vi "GetState.vi"(6 "error in (no error)":errorcluster, 7 "Calibrate?":bool, 8 "IMU Channel":tag="A/I2C", 9 "LIDAR Channel":tag="B/I2C") -> (0 "error out":errorcluster, 1 "Height":dbl, 2 "Angular Velocity":dbl[](array[numeric]), 3 "imu accel":i16[](array[numeric]))   [LabVIEW 2017]
uses:
  <vilib>/Analysis/baseanly.llb/Mean (DBL).vi
  <vilib>/Analysis/NI_AALBase.lvlib
panel:
  out "error out 2":errorcluster
  out "Acceleration":dbl[](array[numeric])
  in  "Acceleration Factor (experimentally determined)":dbl format="%#_13g"
  out "MyRIO Acceleration":dbl[](array[numeric])
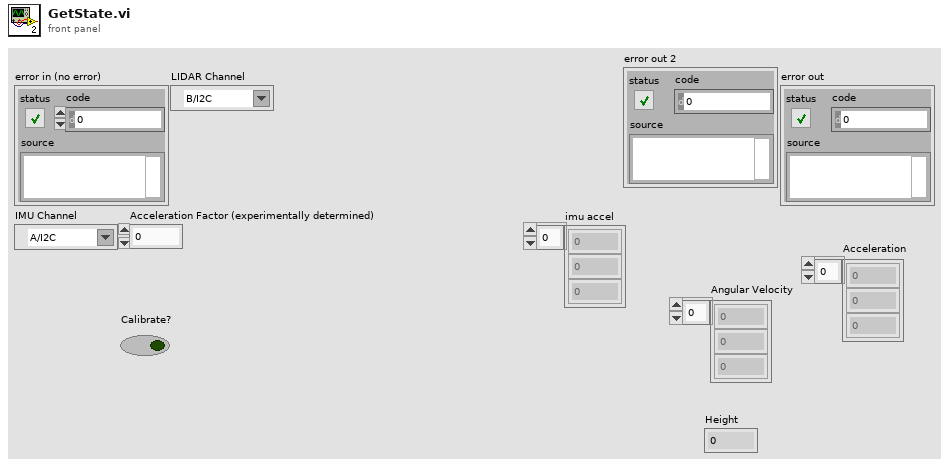
[diagram p1: front panel]
types:
  T1 = cluster{"X-axis":i16, "Y-axis":i16, "Z-axis":i16}
  T2 = cluster{"X-Axis":dbl, "Y-Axis":dbl, "Z-Axis":dbl}
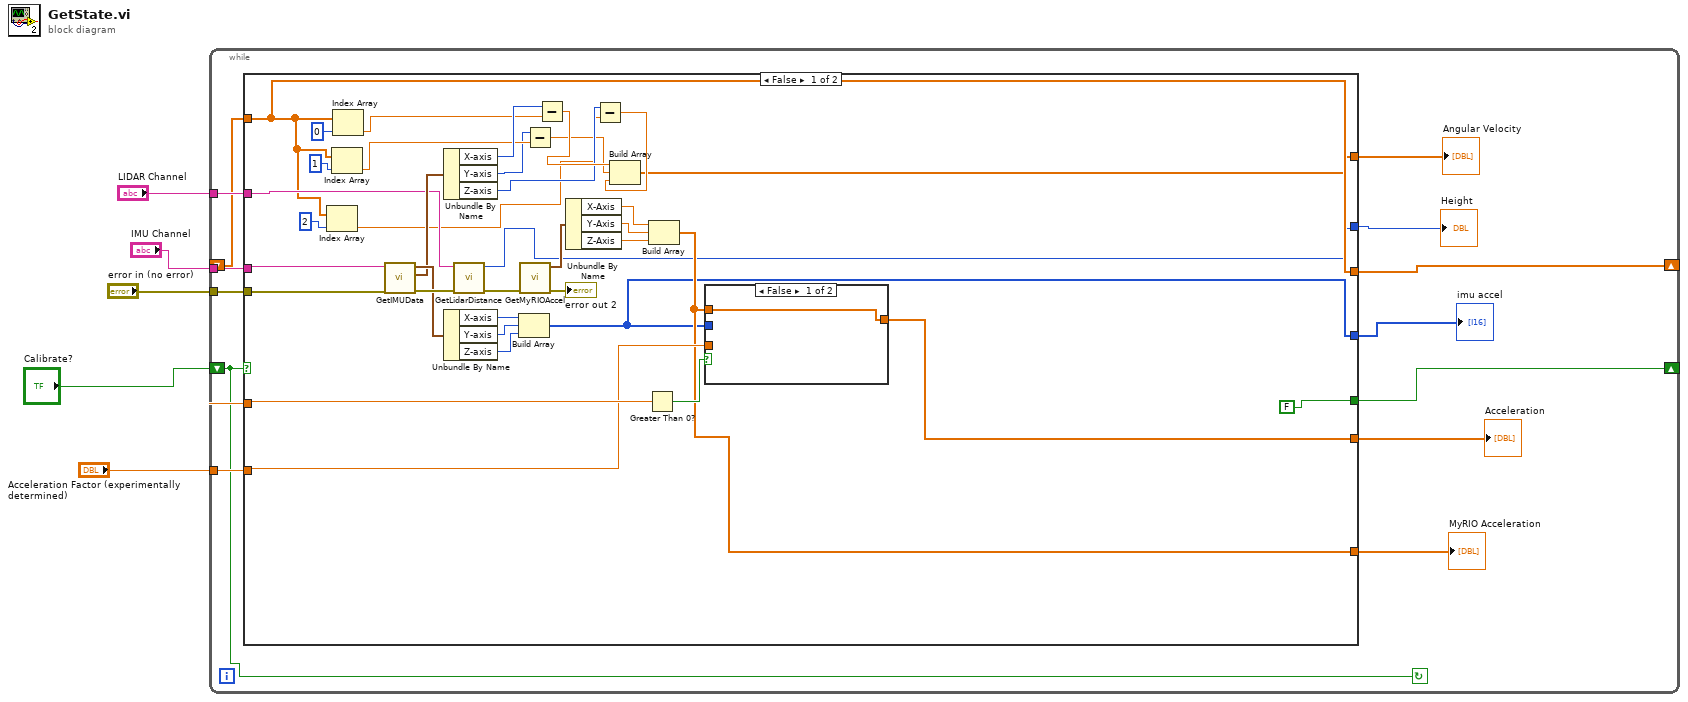
[diagram p0: block diagram]
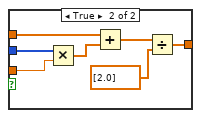
[diagram p2: hidden frame]
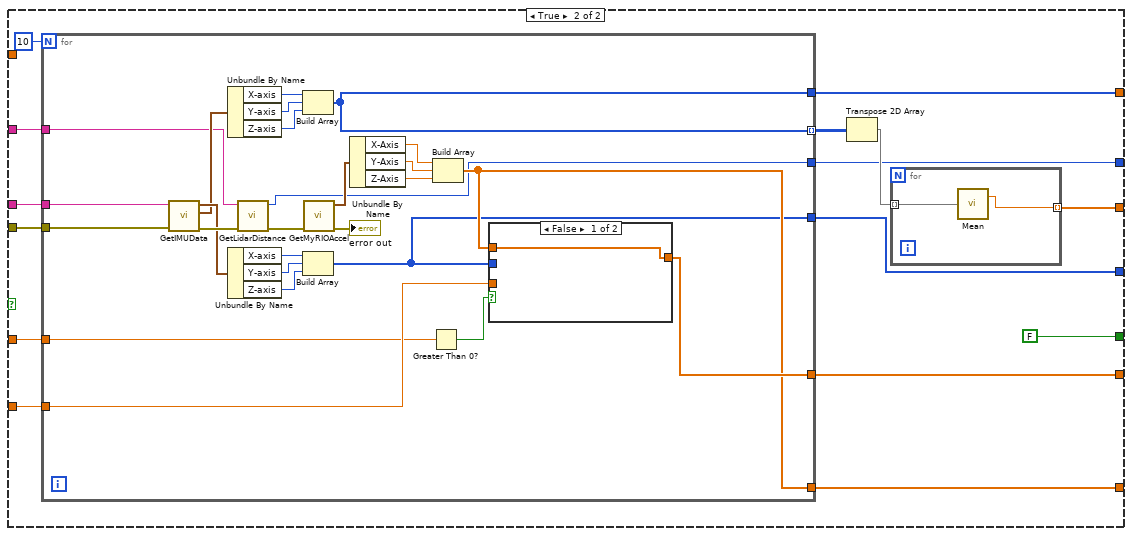
[diagram p3: hidden frame]
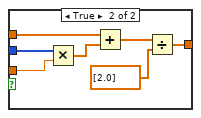
[diagram p4: hidden frame]
diagram:
  n1 = while {
    tunnel: "error in (no error)" -> [w18]
    tunnel: "IMU Channel" -> [w17]
    tunnel: "LIDAR Channel" -> [w16]
    tunnel: "Acceleration Factor (experimentally determined)" -> [w15]
    shift-right: [w14] -> _
    shift-left: "Calibrate?" -> [w13]
    shift-right: [w12] -> _
    shift-left: _ -> [w11]
    stop <- w13 continue-if-true
    n2 = case shown="False" w13 {
      tunnel: w18 -> [w40 w78]
      tunnel: w17 -> [w41 w77]
      tunnel: w16 -> [w42 w76]
      tunnel: w15 -> [w38 w75]
      tunnel: w15 -> [w39 w74]
      tunnel: [FALSE FALSE] -> w14
      tunnel: [w25 w69] -> w12
      tunnel: w11 -> [w25 _]
      tunnel: [w20 w68] -> w10
      tunnel: [w23 w67] -> w9
      tunnel: [w22 w66] -> w8
      tunnel: [w21 w65] -> w7
      tunnel: [w19 w64] -> w6
      frame False {
        n3 = Index Array(array=w25, index=2) -> (element=w28:dbl)
        n4 = Index Array(array=w25, index=1) -> (element=w31:dbl)
        n5 = Index Array(array=w25, index=0) -> (element=w35:dbl)
        n6 = call "GetIMUData.vi"("error in (no error)"=w40, "Channel Name"=w41) -> ("error out"=w55:errorcluster, "GyroData"=w50:T1, "AccelData"=w51:T1)  [unwired: 7 in]
        n7 = Unbundle By Name(w50) -> ("X-axis"=w36:i16, "Y-axis"=w30:i16, "Z-axis"=w29:i16)
        n8 = Unbundle By Name(w51) -> ("X-axis"=w46:i16, "Y-axis"=w45:i16, "Z-axis"=w44:i16)
        n9 = call "GetLidarDistance.vi"("error in"=w55, "Channel Name"=w42) -> ("error out"=w54:errorcluster, "(hi.lo)"=w19:u16)  [unwired: 8 in]
        n10 = Build Array(w46, w45, w44) -> (w21:i16[])
        n11 = call "GetMyRIOAccel.vi"("error in (no error)"=w54) -> ("error out"=→"error out 2":errorcluster, "output cluster"=w52:T2)  [unwired: 9 in]
        n12 = Subtract(x=w30, y=w31) -> (x-y=w27:dbl)
        n13 = Subtract(x=w36, y=w35) -> (x-y=w34:dbl)
        n14 = Unbundle By Name(w52) -> ("X-Axis"=w49:dbl, "Y-Axis"=w48:dbl, "Z-Axis"=w47:dbl)
        n15 = Subtract(x=w29, y=w28) -> (x-y=w26:dbl)
        n16 = Build Array(w34, w27, w26) -> (w20:dbl[])
        n17 = Greater Than 0?(x=w39) -> (x > 0?=w43:bool)
        n18 = Build Array(w49, w48, w47) -> (w22:dbl[])
        n19 = case shown="False" w43 {
          tunnel: w38 -> [_ w63]
          tunnel: w21 -> [_ w62]
          tunnel: w22 -> [w56 w60]
          tunnel: [w56 w57] -> w23
          frame False {
          }
          frame True {
            n20 = Multiply(x=w62, y=w63) -> (x*y=w61:dbl[])
            n21 = Add(x=w60, y=w61) -> (x+y=w59:dbl[])
            n22 = Divide(x=w59, y=dbl[] [2.0]) -> (x/y=w57:dbl[])
          }
        }
      }
      frame True {
        n23 = for {
          N: 10 -> [_]
          tunnel: [w85] -> w72 mode=indexing
          tunnel: w78 -> [w90]
          tunnel: w77 -> [w89]
          tunnel: w76 -> [w88]
          tunnel: w75 -> [w87]
          tunnel: w74 -> [w86]
          tunnel: [w85] -> w68
          tunnel: [w84] -> w67
          tunnel: [w83] -> w66
          tunnel: [w82] -> w65
          tunnel: [w81] -> w64
          n24 = call "GetIMUData.vi"("error in (no error)"=w90, "Channel Name"=w89) -> ("error out"=w106:errorcluster, "GyroData"=w101:T1, "AccelData"=w102:T1)  [unwired: 7 in]
          n25 = Unbundle By Name(w101) -> ("X-axis"=w97:i16, "Y-axis"=w96:i16, "Z-axis"=w95:i16)
          n26 = Unbundle By Name(w102) -> ("X-axis"=w94:i16, "Y-axis"=w93:i16, "Z-axis"=w92:i16)
          n27 = call "GetLidarDistance.vi"("error in"=w106, "Channel Name"=w88) -> ("error out"=w105:errorcluster, "(hi.lo)"=w81:u16)  [unwired: 8 in]
          n28 = Build Array(w97, w96, w95) -> (w85:i16[])
          n29 = Build Array(w94, w93, w92) -> (w82:i16[])
          n30 = call "GetMyRIOAccel.vi"("error in (no error)"=w105) -> ("error out"=→"error out":errorcluster, "output cluster"=w103:T2)  [unwired: 9 in]
          n31 = Unbundle By Name(w103) -> ("X-Axis"=w100:dbl, "Y-Axis"=w99:dbl, "Z-Axis"=w98:dbl)
          n32 = Greater Than 0?(x=w86) -> (x > 0?=w91:bool)
          n33 = Build Array(w100, w99, w98) -> (w83:dbl[])
          n34 = case shown="False" w91 {
            tunnel: w87 -> [_ w114]
            tunnel: w82 -> [_ w113]
            tunnel: w83 -> [w107 w111]
            tunnel: [w107 w108] -> w84
            frame False {
            }
            frame True {
              n35 = Multiply(x=w113, y=w114) -> (x*y=w112:dbl[])
              n36 = Add(x=w111, y=w112) -> (x+y=w110:dbl[])
              n37 = Divide(x=w110, y=dbl[] [2.0]) -> (x/y=w108:dbl[])
            }
          }
        }
        n38 = Transpose 2D Array(2D array=w72) -> (transposed array=w71:i16[][])
        n39 = for {
          tunnel: w71 -> [w80] mode=indexing
          tunnel: [w79] -> w69 mode=indexing
          n40 = call-poly <vilib>:"Mean.vi"("X"=w80) -> ("mean"=w79:dbl)  [unwired: 1 out]
        }
      }
    }
    "Angular Velocity" <- w10
    "Acceleration" <- w9
    "MyRIO Acceleration" <- w8
    "imu accel" <- w7
    "Height" <- w6
  }
